vi "Read Component Product Name -_ Unique Name.vi"(8 "error in (no error)":errorcluster, 11 "Build Analyzer in":refnum<class "Build Analyzer.lvclass">) -> (0 "error out":errorcluster, 2 "Component Product Name -> Unique Name":variant, 3 "Build Analyzer out":refnum<class "Build Analyzer.lvclass">)   [LabVIEW 2017, in "CL_G3_VIComponentBuilder.lvlib" / "Build Analyzer.lvclass"]
uses:
  Build Analyzer.lvclass
  Build Analyzer.lvclass/Build Analyzer.ctl
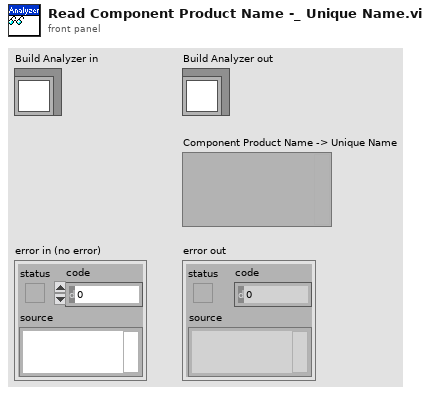
[diagram p1: front panel]
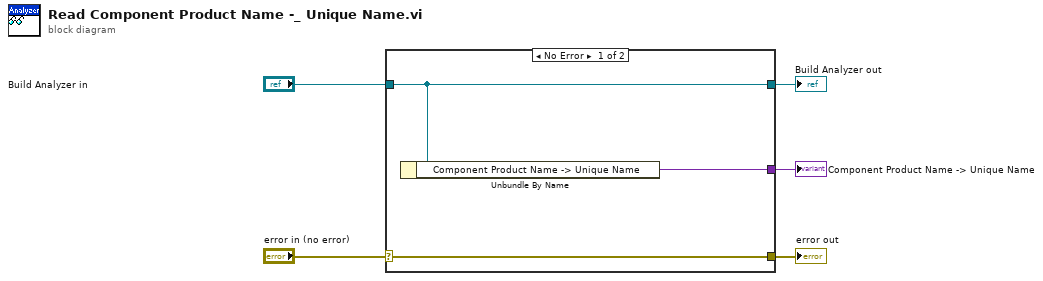
[diagram p0: block diagram]
diagram:
  n1 = case shown="No Error" "error in (no error)" {
    selector: "error in (no error)" -> [w8 w9]
    tunnel: [w8 w9] -> w4
    tunnel: [w7 w10] -> w2
    tunnel: "Build Analyzer in" -> [w7 w10]
    tunnel: [w6 _] -> w1
    frame No Error {
      n2 = Unbundle By Name(w7) -> ("Component Product Name -> Unique Name"=w6:variant)
    }
    frame Error {
    }
  }
  "error out" <- w4
  "Build Analyzer out" <- w2
  "Component Product Name -> Unique Name" <- w1
